vi "Set_DL.vi"(8 "error in (no error)":errorcluster, 11 "Control-Server in":refnum<class "Control-Server.lvclass">) -> (0 "error out":errorcluster, 3 "Control-Server out":refnum<class "Control-Server.lvclass">)   [LabVIEW 2019, in "Control-Server.lvclass"]
uses:
  Control-Server.lvclass
  Config/config_names_def.ctl
  Delay Line/DelayLineSimulation/DLEmulate.lvclass
  C:/Users/elysium/Documents/dev/TRANCON/Classes/Delay Line/DelayLine.lvclass
  Delay Line/DelayLineLS4/DLLS4.lvclass
  Delay Line/DelayLineOwis/DLOwis.lvclass
  dependecies/ControlsVIs/Clusters-def/UserEvent.ctl
  dependecies/ControlsVIs/Clusters-def/Message types.ctl
  Message/Message.lvclass
  Message/Message.lvclass/Message.ctl
  GeneralFunctionality/GeneralFunctionality.lvclass/GeneralFunctionality.ctl
  Control-Server.lvclass/Control-Server.ctl
  Delay Line/DelayLine.lvclass
  C:/Users/elysium/Documents/dev/TRANCON/Classes/GeneralFunctionality/GeneralFunctionality.lvclass
  Config/Config.lvclass
  GeneralFunctionality/GeneralFunctionality.lvclass
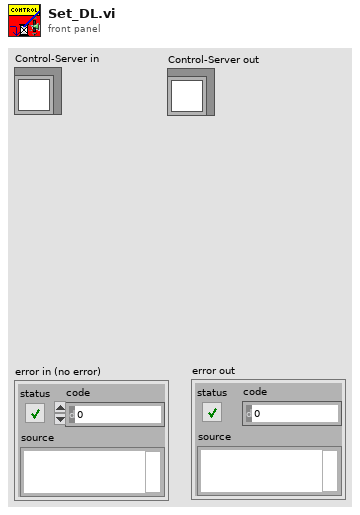
[diagram p1: front panel]
types:
  T1 = typedef "Config.lvclass/config_names_def.ctl" = string
  T2 = typedef "Message types.ctl" = string
  T3 = typedef "UserEvent.ctl" = cluster{"command":string, "data":variant}
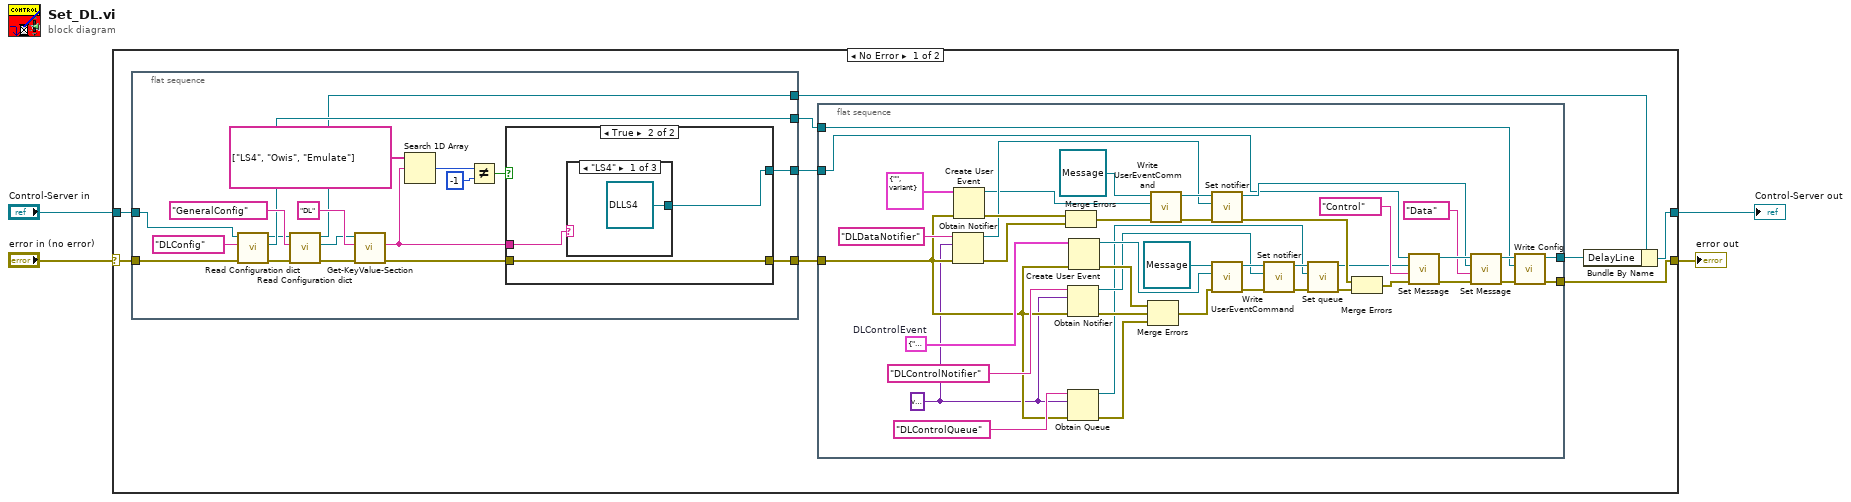
[diagram p0: block diagram]
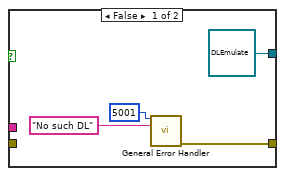
[diagram p2: hidden frame]
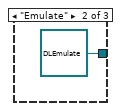
[diagram p3: hidden frame]
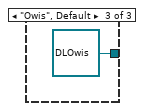
[diagram p4: hidden frame]
diagram:
  n1 = case shown="No Error" "error in (no error)" {
    selector: "error in (no error)" -> [w8 w85]
    tunnel: "Control-Server in" -> [w9 w86]
    tunnel: [w7 w85] -> w2
    tunnel: [w6 w86] -> w1
    frame No Error {
      n2 = flat-sequence {
        tunnel: w9 -> [w29]
        tunnel: w8 -> [w28]
        tunnel: [w30] -> w11
        tunnel: [w16] -> w12
        tunnel: [w24] -> w13
        tunnel: [w15] -> w5
        frame #0 {
          n3 = call "Read Configuration dict.vi"("error in (no error)"=w28, "Config Name"=T1 "DLConfig", "Control in"=w29) -> ("error out"=w18:errorcluster, "Config"=w30:refnum<class "Config.lvclass">, "Control out"=w19:refnum<class "Control-Server.lvclass">)  [unwired: 6 in]
          n4 = call "Read Configuration dict.vi"("error in (no error)"=w18, "Config Name"=T1 "GeneralConfig", "Control in"=w19) -> ("error out"=w17:errorcluster, "Config"=w14:refnum<class "Config.lvclass">, "Control out"=w15:refnum<class "Control-Server.lvclass">)  [unwired: 6 in]
          n5 = call-dynamic "Get-KeyValue-Section.vi"("error in (no error)"=w17, "Section"="DL", "Config in"=w14) -> ("error out"=w21:errorcluster, "Value"=w20:string)  [unwired: 6 in, 1 out]
          n6 = Search 1D Array(1D array=string[] ["LS4", "Owis", "Emulate"], element=w20) -> (index of element=w26:i32)  [unwired: 1 in]
          n7 = Not Equal?(x=w26, y=-1) -> (x != y?=w25:bool)
          n8 = case shown="True" w25 {
            tunnel: [w34 w38] -> w16
            tunnel: [refnum<class "DLEmulate.lvclass"> refnum ("DLEmulate.lvclass") w39] -> w24
            tunnel: w21 -> [_ w38]
            tunnel: w20 -> [_ w37]
            frame False {
              n9 = call <vilib>:"General Error Handler.vi"("[error code] (0)"=5001 ("code"), "[error source] (\" \")"="No such DL" ("String to Prepend to source (\"\")")) -> ("error out"=w34:errorcluster)  [unwired: 9 in, 4 out]
            }
            frame True {
              n10 = case shown="\"LS4\"" w37 {
                tunnel: [refnum<class "DLLS4.lvclass"> refnum ("DelayLineLS4.lvclass") refnum<class "DLEmulate.lvclass"> refnum ("DelayLineEmulate.lvclass") refnum<class "DLOwis.lvclass"> refnum ("DelayLineOwis.lvclass")] -> w39
                frame "LS4" {
                }
                frame "Emulate" {
                }
                frame "Owis", Default {
                }
              }
            }
          }
        }
      }
      n11 = flat-sequence {
        tunnel: w11 -> [w45]
        tunnel: [w84] -> w10
        tunnel: [w83] -> w7
        tunnel: w12 -> [w48]
        tunnel: w13 -> [w44]
        frame #0 {
          w43 = variant
          w78 = cluster{"command":string, "data":variant} {"command"="", "data"=variant}  # DLControlEvent
          n12 = Obtain Notifier(name (unnamed)="DLDataNotifier" ("nom (aucun)"), notification data type=w43, error in (no error)=w48) -> (notifier out=w59:refnum<notifier>, error out=w63:errorcluster)  [unwired: 1 in, 1 out]
          n13 = Create User Event(user event datatype=T3 {"command"="", "data"=variant} ("DLDataEvent"), error in=w48) -> (user event=w58:refnum<user-event>, error out=w64:errorcluster)
          n14 = Merge Errors(w64, w63) -> (w62:errorcluster)
          n15 = Obtain Notifier(name (unnamed)="DLControlNotifier" ("nom (aucun)"), notification data type=w43, error in (no error)=w48) -> (notifier out=w74:refnum<notifier>, error out=w75:errorcluster)  [unwired: 1 in, 1 out]
          n16 = Obtain Queue(name (unnamed)="DLControlQueue", element data type=w43, error in (no error)=w48) -> (queue out=w50:refnum<queue>, error out=w49:errorcluster)  [unwired: 2 in, 1 out]
          n17 = Create User Event(user event datatype=w78, error in=w48) -> (user event=w80:refnum<user-event>, error out=w76:errorcluster)
          n18 = Merge Errors(w76, w75, w49) -> (w73:errorcluster)
          n19 = call "Write UserEventCommand.vi"("error in (no error)"=w62, "UserEventCommand"=w58, "Message en entrée"=refnum<class "Message.lvclass"> refnum ("Message.lvclass")) -> ("error out"=w61:errorcluster, "Message en sortie"=w60:refnum<class "Message.lvclass">)  [unwired: 7 in]
          n20 = call "Set notifier.vi"("error in (no error)"=w61, "notifier"=w59, "Message en entrée"=w60) -> ("error out"=w56:errorcluster, "Message en sortie"=w54:refnum<class "Message.lvclass">)  [unwired: 7 in]
          n21 = call "Write UserEventCommand.vi"("error in (no error)"=w73, "UserEventCommand"=w80, "Message en entrée"=refnum<class "Message.lvclass"> refnum ("Message.lvclass")) -> ("error out"=w77:errorcluster, "Message en sortie"=w81:refnum<class "Message.lvclass">)  [unwired: 7 in]
          n22 = call "Set notifier.vi"("error in (no error)"=w77, "notifier"=w74, "Message en entrée"=w81) -> ("error out"=w51:errorcluster, "Message en sortie"=w52:refnum<class "Message.lvclass">)  [unwired: 7 in]
          n23 = call "Set queue.vi"("error in (no error)"=w51, "queue"=w50, "Message in"=w52) -> ("error out"=w47:errorcluster, "Message out"=w46:refnum<class "Message.lvclass">)  [unwired: 7 in]
          n24 = Merge Errors(w56, w47) -> (w55:errorcluster)
          n25 = call "Set Message.vi"("error in (no error)"=w55, "Message type"=T2 "Control", "Message.lvclass"=w46, "GeneralFunctionality en entrée"=w44) -> ("error out"=w69:errorcluster, "GeneralFunctionality en sortie"=w68:refnum<class "DelayLine.lvclass">)  [unwired: 6 in]
          n26 = call "Set Message.vi"("error in (no error)"=w69, "Message type"=T2 "Data", "Message.lvclass"=w54, "GeneralFunctionality en entrée"=w68) -> ("error out"=w67:errorcluster, "GeneralFunctionality en sortie"=w66:refnum<class "DelayLine.lvclass">)  [unwired: 6 in]
          n27 = call "Write Config.vi"("error in (no error)"=w67, "Config.lvclass"=w45, "GeneralFunctionality en entrée"=w66) -> ("error out"=w83:errorcluster, "GeneralFunctionality en sortie"=w84:refnum<class "DelayLine.lvclass">)  [unwired: 7 in]
        }
      }
      n28 = Bundle By Name(cluster=w5, "DelayLine"=w10) -> (w6:refnum<class "Control-Server.lvclass">)
    }
    frame Error {
    }
  }
  "error out" <- w2
  "Control-Server out" <- w1
